vi "Write Stop.vi"(8 "error in (no error)":errorcluster, 10 "stop":bool, 11 "Thread in":refnum<class "Thread.lvclass">) -> (0 "error out":errorcluster, 3 "Thread out":refnum<class "Thread.lvclass">)   [LabVIEW 2017, in "DSF Core.lvlib" / "Thread.lvclass"]
uses:
  Thread.lvclass
  Thread.lvclass/Thread.ctl
  LabVIEW-Memory/Source/Classes/Pointer/Write Bool.vi
  LabVIEW-Memory/Source/Classes/Pointer/Pointer.lvclass
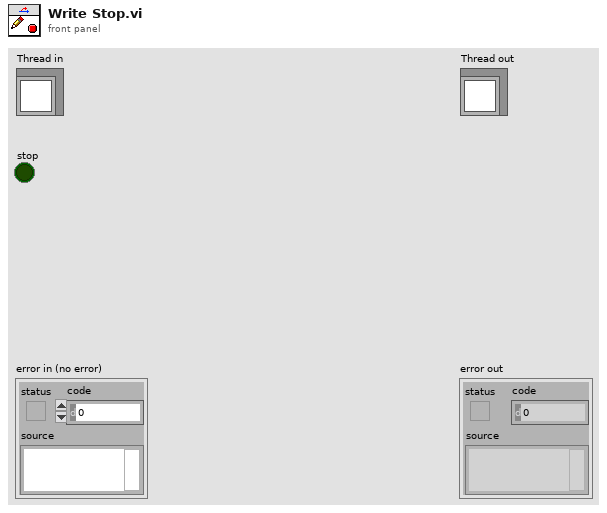
[diagram p1: front panel]
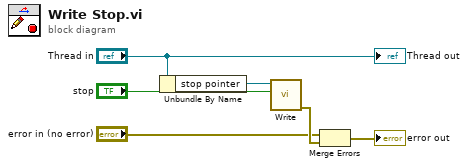
[diagram p0: block diagram]
diagram:
  n1 = Unbundle By Name("Thread in") -> ("stop pointer"=w6:refnum<class "Pointer.lvclass">)
  n2 = call-poly "Write.vi"("value"="stop", "Pointer in"=w6) -> ("error out"=w3:errorcluster)  [unwired: 6 in, 3 out]
  n3 = Merge Errors("error in (no error)", w3) -> (→"error out":errorcluster)
  "Thread out" <- "Thread in"
